vi "Find Ring BAP7.vi"(11 "BrickReference in":T2) -> (2 "Motor Out":cluster{"Port":T1, "Port":T1}={"Port"=1, "Port"=3} {"Port" items=["Port A", "Port B", "Port C", "Port D"]; "Port" items=["Port A", "Port B", "Port C", "Port D"]}, 3 "BrickReference Out":T2)   [LabVIEW 2014]
doc: "Find Ring BAP7\n\nKeeps moving forward until it senses the change in floor color from black to white to black again. At that point it plays a note, indicating that it has entered the ring and then moves slowly to the center.\n\nBeverly Abadines\nPHY 350\nBAP7"
uses:
  <vilib>/NXT/Subs/LVHSConnector.ctl
  <vilib>/NXT/LegoClasses/BrickReference/BrickReference.lvclass
  <vilib>/NXT/Block Support/NXT_OutputPort.ctl
  <vilib>/NXT/Block Support/NXT_InputPort.ctl
  <vilib>/NXT/NXTIO Xnodes/NXTIONodeSubVIs/NXTMotorSteeringOn.vi
  <vilib>/NXT/Dual Mode Library/Display/drawNumber.vi
  <vilib>/NXT/Dual Mode Library/Sound/PlayC.vi
  <vilib>/NXT/NXTIO Xnodes/AddressXNode/NXTIOAddress.xnode
  <vilib>/NXT/NXTIO Xnodes/NXTIOXNode/NXTIO.xnode
panel:
  out "Color Dif.":i16
  # "Find  Ring"
  # "Beverly Abadines\nPhys 350\nP7"
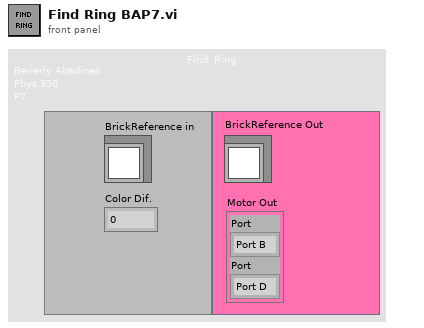
[diagram p1: front panel]
types:
  T1 = typedef "NXT_OutputPort.ctl" = u8
  T2 = typedef "LVHSConnector.ctl" = refnum<class "BrickReference.lvclass">
  T3 = typedef "NXT_InputPort.ctl" = u32
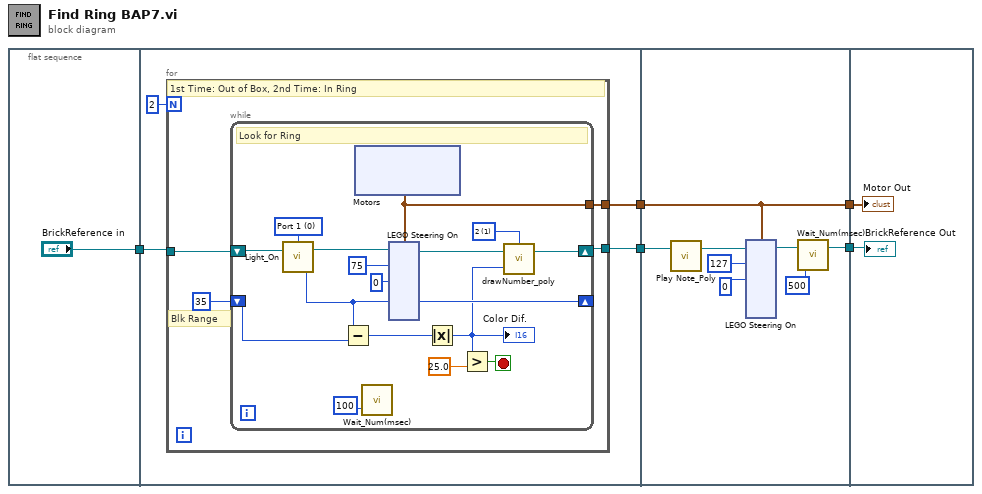
[diagram p0: block diagram]
diagram:
  n1 = flat-sequence {
    tunnel: ["BrickReference in"] -> w5
    tunnel: w5 -> [w9]
    tunnel: [w8] -> w4
    tunnel: [w7] -> w2
    tunnel: w4 -> [w47]
    tunnel: [w41] -> w3
    tunnel: w2 -> [w44]
    tunnel: [w44] -> w1
    tunnel: w3 -> [w57]
    tunnel: w1 -> [w56]
    frame #0 {
    }
    frame #1 {
      n2 = for {
        N: 2 -> [_]
        tunnel: w9 -> [w14]
        tunnel: [w12] -> w8
        tunnel: [w11] -> w7
        # "Blk Range"
        # "1st Time: Out of Box, 2nd Time: In Ring"
        n3 = while {
          shift-right: [w23] -> _
          shift-left: i16 35 ("Scaled Value") -> [w22]
          shift-right: [w17] -> w12
          shift-left: w14 -> [w30]
          tunnel: [w15] -> w11
          stop <- w27 stop-if-true
          w20 = i16 1 items=["1", "2", "3", "4", "5", "6", "7", "8", "9", "10", "11", "12"] ("Line")
          w29 = T3 0 items=["Port 1", "Port 2", "Port 3", "Port 4"] ("Port (Port 3)")
          # "Look for Ring"
          n4 = call <vilib>:"Light_On.vi"("NXT/EV3"=w30, "Port (Port 3)"=w29) -> ("Scaled Value"=w23:i16, "NXT/EV3"=w26:T2)  [unwired: 1 in]
          n5 = Subtract(x=w23, y=w22) -> (x-y=w21:i16)
          n6 = xnode "Motors"() -> ("Motor"=w15:cluster{"Port":T1, "Port":T1})
          n7 = call <vilib>:"Wait_Num(msec).vi"("Time (100 msec)"=u32 100) -> ()  [unwired: 3 in, 1 out]
          n8 = xnode "LEGO Steering On"("Steering 1"=0, "Power 1"=75, "Motors"=w15, "NXT/EV3"=w26) -> ("NXT/EV3"=w18:T2)
          n9 = Absolute Value(x=w21) -> (abs(x)=w19:i16)
          "Color Dif." <- w19
          n10 = Greater?(x=w19, y=25.0) -> (0:w27:bool)
          n11 = call-poly <vilib>:"drawNumber_poly.vi"("number"=w19, "NXT/EV3"=w18, "Line"=w20) -> ("NXT/EV3"=w17:T2)  [unwired: 1 in]
        }
      }
    }
    frame #2 {
      n12 = call-poly <vilib>:"Play Note_Poly.vi"("NXT/EV3"=w47) -> ("NXT/EV3"=w46:T2)  [unwired: 3 in]
      n13 = xnode "LEGO Steering On"("Steering 1"=0, "Power 1"=127, "Motors"=w44, "NXT/EV3"=w46) -> ("NXT/EV3"=w42:T2)
      n14 = call <vilib>:"Wait_Num(msec).vi"("Time (100 msec)"=u32 500, "NXT/EV3"=w42) -> ("NXT/EV3"=w41:T2)  [unwired: 2 in]
    }
    frame #3 {
      "BrickReference Out" <- w57
      "Motor Out" <- w56
    }
  }
